vi "弧度至角度1D（单位）vi.vi"(1 "radians":dbl[unit][](array[numeric])) -> (0 "degree":dbl[unit][](array[numeric]))   [LabVIEW 2012, in "几何工具.lvlib"]
doc: "功能：\n\n一维数组弧度转换为角度。\n\n输入：弧度。\n\n输出：角度，单位为度。\n\ncsxcs_366创建。"
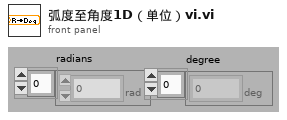
[diagram p1: front panel]
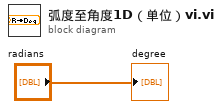
[diagram p0: block diagram]
diagram:
  "degree" <- "radians"
